vi "Tip touchdown.vi"(10 "Z SetPoint":dbl format="%#_6p") -> ()   [LabVIEW 2013]
doc: "Touch down tip on sample surface. The Z Set point determines the loading force on tip when it engaged on sample surface."
panel:
  out "error out":errorcluster
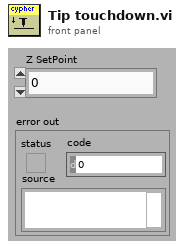
[diagram p1: front panel]
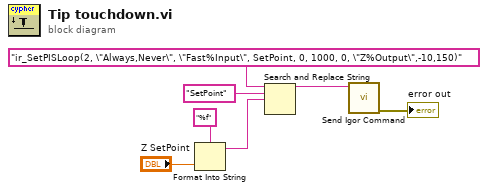
[diagram p0: block diagram]
diagram:
  n1 = Format Into String(format string="%f", "Z SetPoint") -> (resulting string=w4:string)  [unwired: 2 in, 1 out]
  n2 = Search and Replace String(input string="ir_SetPISLoop(2, \"Always,Never\", \"Fast%Input\", SetPoint, 0, 1000, 0, \"Z%Output\",-10,150)", search string="SetPoint", replace string=w4) -> (result string=w1:string)  [unwired: 1 in, 7 out]
  n3 = call "Send Igor Command.vi"("Command"=w1) -> ("error out"=→"error out":errorcluster)  [unwired: 7 in, 2 out]
